vi "Write Sequence Name.vi"(8 "error in (no error)":errorcluster, 10 "Sequence Name":string, 11 "SequenceNode in":refnum<class "SequenceNode.lvclass">) -> (0 "error out":errorcluster, 3 "SequenceNode out":refnum<class "SequenceNode.lvclass">)   [LabVIEW 2015, in "SequenceNode.lvclass"]
uses:
  SequenceNode.lvclass
  SequenceNode.lvclass/SequenceNode.ctl
  Prototype/classes/Sequence/Config/Sequence Config.lvclass
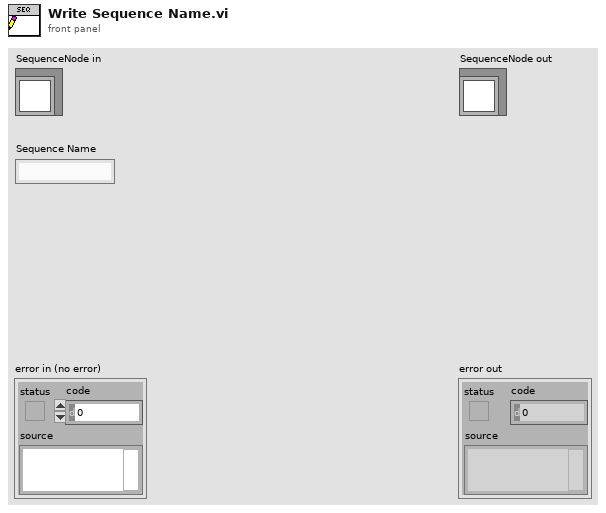
[diagram p1: front panel]
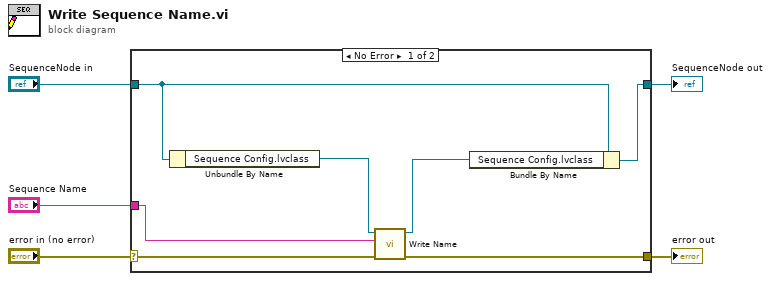
[diagram p0: block diagram]
diagram:
  n1 = case shown="No Error" "error in (no error)" {
    selector: "error in (no error)" -> [w12 w13]
    tunnel: [w9 w13] -> w4
    tunnel: [w11 w14] -> w2
    tunnel: "SequenceNode in" -> [w10 w14]
    tunnel: "Sequence Name" -> [w6 _]
    frame No Error {
      n2 = Unbundle By Name(w10) -> ("Sequence Config.lvclass"=w8:refnum<class "Sequence Config.lvclass">)
      n3 = call-dynamic "Write Name.vi"("error in (no error)"=w12, "Name"=w6, "Sequence in"=w8) -> ("error out"=w9:errorcluster, "Sequence out"=w7:refnum<class "Sequence Config.lvclass">)  [unwired: 7 in]
      n4 = Bundle By Name(cluster=w10, "Sequence Config.lvclass"=w7) -> (w11:refnum<class "SequenceNode.lvclass">)
    }
    frame Error {
    }
  }
  "error out" <- w4
  "SequenceNode out" <- w2
